vi "Parse (Gyro Stabilized Acceleration, Angular Rate, And Magnetometer Vectors).vi"(7 "Message In":string) -> (4 "Gyro Stabilized Acceleration Vector":sgl[](array[numeric]), 6 "Gyro Stabilized Angular Rate Vector":sgl[](array[numeric]), 8 "Gyro Stabilized Magnetometer Vetor":sgl[](array[numeric]), 15 "Timer":u32)   [LabVIEW 2012, in "MicroStrain 3DM-GXx.lvlib"]
doc: "Parse the data from the 0xD2 message into the Gyro Stabilized Acceleration Vector (m/s^2), Gyro Stabilized Angular Rate Vector (rad/s), and the Gyro Stabilized Magnetometer Vector (G)."
uses:
  <instrlib>/MicroStrain 3DM-GXx/MicroStrain 3DM-GXx.lvlib
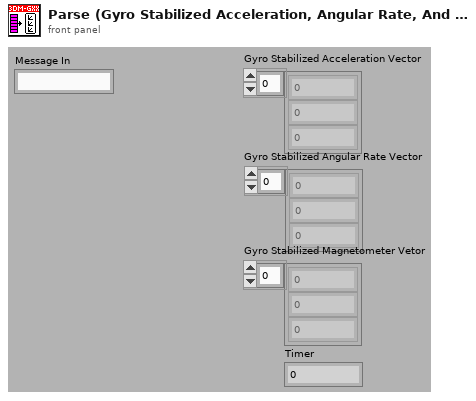
[diagram p1: front panel]
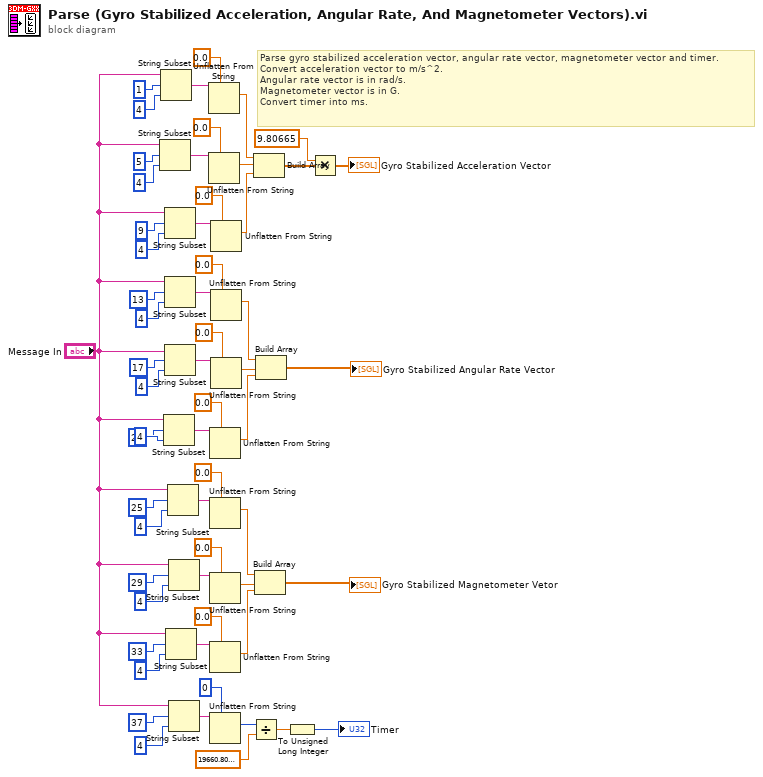
[diagram p0: block diagram]
diagram:
  # "Parse gyro stabilized acceleration vector, angular rate vector, magnetometer vector and timer.\nConvert acceleration vector to m/s^2.\nAngular rate vector is in rad/s.\nMagnetometer vector is in G.\nConvert timer into ms."
  n1 = String Subset(string="Message In", offset (0)=5, length (rest)=4 ("length (rest)")) -> (substring=w54:string)
  n2 = String Subset(string="Message In", offset (0)=1, length (rest)=4 ("length (rest)")) -> (substring=w57:string)
  n3 = String Subset(string="Message In", offset (0)=21, length (rest)=4 ("length (rest)")) -> (substring=w31:string)
  n4 = String Subset(string="Message In", offset (0)=9, length (rest)=4 ("length (rest)")) -> (substring=w49:string)
  n5 = String Subset(string="Message In", offset (0)=13, length (rest)=4 ("length (rest)")) -> (substring=w39:string)
  n6 = String Subset(string="Message In", offset (0)=17, length (rest)=4 ("length (rest)")) -> (substring=w34:string)
  n7 = String Subset(string="Message In", offset (0)=33, length (rest)=4 ("length (rest)")) -> (substring=w18:string)
  n8 = String Subset(string="Message In", offset (0)=25, length (rest)=4 ("length (rest)")) -> (substring=w26:string)
  n9 = String Subset(string="Message In", offset (0)=29, length (rest)=4 ("length (rest)")) -> (substring=w23:string)
  n10 = String Subset(string="Message In", offset (0)=37, length (rest)=4 ("length (rest)")) -> (substring=w45:string)
  n11 = Unflatten From String(type=sgl 0.0, binary string=w57) -> (value=w11:sgl)  [unwired: 3 in, 2 out]
  n12 = Unflatten From String(type=sgl 0.0, binary string=w54) -> (value=w12:sgl)  [unwired: 3 in, 2 out]
  n13 = Unflatten From String(type=sgl 0.0, binary string=w31) -> (value=w6:sgl)  [unwired: 3 in, 2 out]
  n14 = Unflatten From String(type=sgl 0.0, binary string=w26) -> (value=w3:sgl)  [unwired: 3 in, 2 out]
  n15 = Unflatten From String(type=sgl 0.0, binary string=w23) -> (value=w4:sgl)  [unwired: 3 in, 2 out]
  n16 = Unflatten From String(type=sgl 0.0, binary string=w18) -> (value=w2:sgl)  [unwired: 3 in, 2 out]
  n17 = Unflatten From String(type=u32 0, binary string=w45) -> (value=w44:u32)  [unwired: 3 in, 2 out]
  n18 = Unflatten From String(type=sgl 0.0, binary string=w49) -> (value=w10:sgl)  [unwired: 3 in, 2 out]
  n19 = Unflatten From String(type=sgl 0.0, binary string=w39) -> (value=w8:sgl)  [unwired: 3 in, 2 out]
  n20 = Unflatten From String(type=sgl 0.0, binary string=w34) -> (value=w7:sgl)  [unwired: 3 in, 2 out]
  n21 = Divide(x=w44, y=sgl 19660.8) -> (x/y=w42:sgl)
  n22 = Build Array(w11, w12, w10) -> (w13:sgl[])
  n23 = Build Array(w3, w4, w2) -> (→"Gyro Stabilized Magnetometer Vetor":sgl[])
  n24 = Build Array(w8, w7, w6) -> (→"Gyro Stabilized Angular Rate Vector":sgl[])
  n25 = To Unsigned Long Integer(number=w42) -> (unsigned 32bit integer=→"Timer":u32)
  n26 = Multiply(x=9.80665, y=w13) -> (x*y=→"Gyro Stabilized Acceleration Vector":dbl[])
